vi "Write1000.vi"() -> ()   [LabVIEW 2015]
uses:
  <vilib>/Platform/TimedLoop/XDataNode/timing_clust.ctl
  <vilib>/Platform/TimedLoop/XDataNode/nitl_modes.ctl
  <vilib>/Platform/TimedLoop/XDataNode/wakeup.ctl
  <vilib>/platform/TimedLoop/XDataNode/XDataNode.xnode
  <vilib>/Platform/TimedLoop/XDataNode/XDNodeRunTimeDep.lvlib
panel:
  out "floor(x/y)":dbl
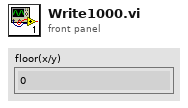
[diagram p1: front panel]
types:
  T1 = typedef "XDNodeRunTimeDep.lvlib/timing_clust.ctl" = cluster{"Expected End [f-1]":u64, "Actual End [f-1]":u64, "Finished Late? [f-1]":bool, "Expected End [i-1]":u64, "Actual End [i-1]":u64, "Finished Late? [i-1]":bool, "Expected Start [i]":u64, "Actual Start [i]":u64, "Expected Start [f]":u64, "Actual Start [f]":u64, "Source Name":string, "Structure Name":string, "Period":i64, "Deadline":i64, "Offset":i64, "Start":i64, "Priority":i32, "Timeout":i32, "Mode":T2, "Wakeup Reason":T3, "Error":errorcluster, "Source Type":string, "Secondary Source Type":string, "Global End Time":u64, "Global Start Time":u64, "Frame Duration":u64, "Iteration Duration":u64, "Assigned CPU":i32, "I/O Scan Engine Mode":u32}
  T2 = typedef "XDNodeRunTimeDep.lvlib/nitl_modes.ctl" = enum32{"No Change", "Process missed periods, maintain original phase", "Discard missed periods, maintain original phase", "Process missed periods, ignore original phase", "Discard missed periods, ignore original phase"}
  T3 = typedef "XDNodeRunTimeDep.lvlib/wakeup.ctl" = enum32{"Normal", "Aborted", "Asynchronous wakeup", "Timing source error", "Timed loop error", "Timeout"}
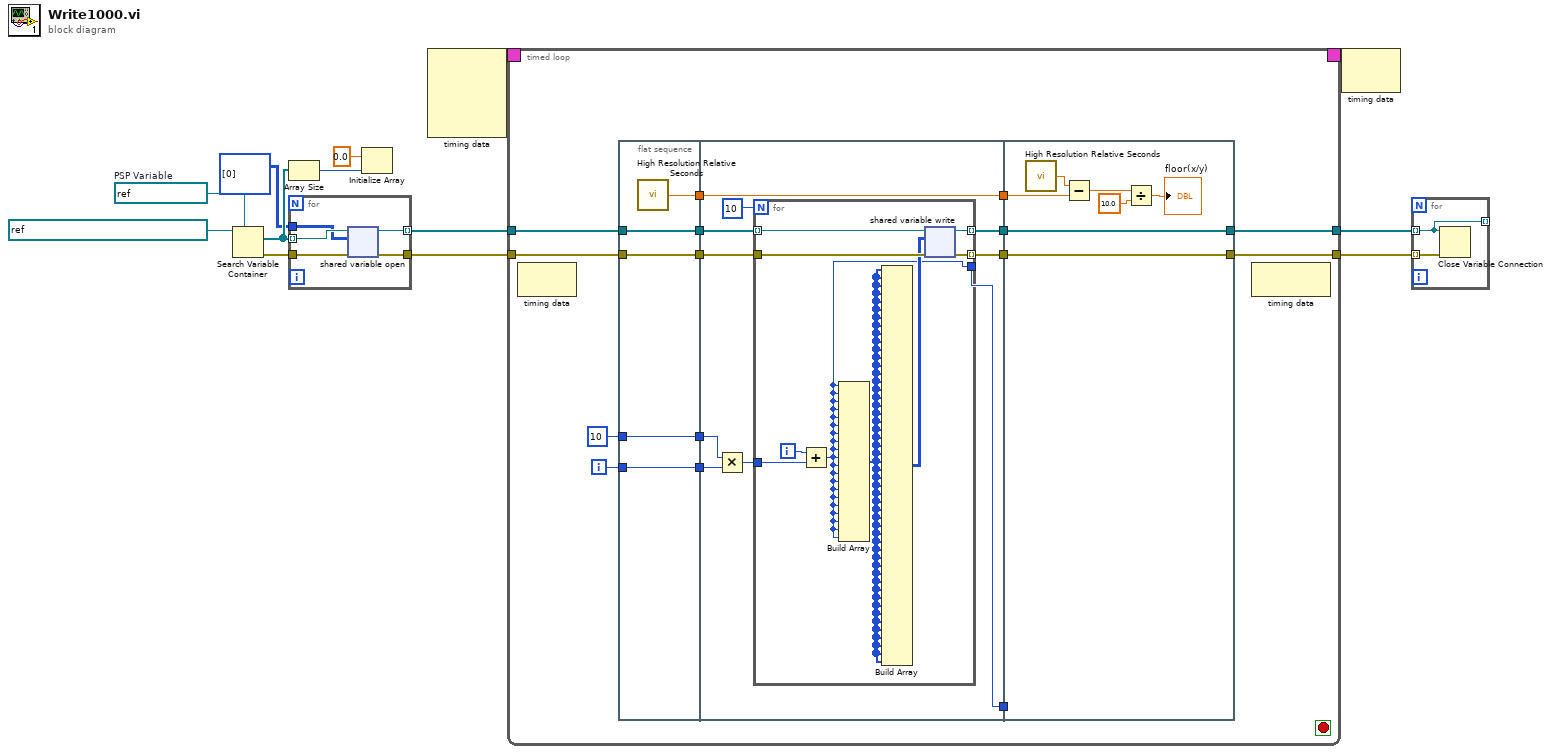
[diagram p0: block diagram]
diagram:
  w13 = refnum<k21> refnum  # PSP Variable
  n1 = Search Variable Container(7:w13, 11:refnum<k21> "ni.var.psp://localhost/Lib1000" ("container refnum in")) -> (0:w11:errorcluster, 2:w7:refnum<k21>[])  [unwired: 4 in, 1 out]
  n2 = Array Size(array=w7) -> (size(s)=w6:i32)
  n3 = for {
    tunnel: w7 -> [w18] mode=indexing
    tunnel: w11 -> [w17]
    tunnel: [w16] -> w3 mode=indexing
    tunnel: [w15] -> w8
    tunnel: i32[][] [[0]] ("appended array") -> [w14]
    n4 = shared-variable-open(w18, w17, w14) -> (w16:refnum<k21>, w15:errorcluster)  [unwired: 1 in]
  }
  n5 = Initialize Array(0.0 ("element"), w6) -> ()  [unwired: 1 out]
  n6 = node-c288() -> (w10:T1)  [unwired: 4 in]
  n7 = timed-loop {
    timing: w10 -> [_]
    timing-out: [_] -> w9
    tunnel: w3 -> [w33]
    tunnel: w8 -> [w32]
    tunnel: [w28] -> w4
    tunnel: [w29] -> w2
    i -> [w31]
    stop <- _ stop-if-true
    n8 = node-c288() -> ()  [unwired: 1 in, 1 out]
    n9 = flat-sequence {
      tunnel: 10 ("x") -> [w35]
      tunnel: w31 -> [w36]
      tunnel: w32 -> [w37]
      tunnel: w33 -> [w38]
      tunnel: [w38] -> w25
      tunnel: [w37] -> w24
      tunnel: [w36] -> w23
      tunnel: [w35] -> w22
      tunnel: [w34] -> w20
      tunnel: [w43] -> w27
      tunnel: [w42] -> w26
      tunnel: w25 -> [w48]
      tunnel: w24 -> [w47]
      tunnel: w23 -> [w46]
      tunnel: w22 -> [w45]
      tunnel: [w39] -> w21
      tunnel: w20 -> [w39]
      tunnel: [w41] -> w19
      tunnel: [w63] -> w28
      tunnel: [w64] -> w29
      tunnel: w27 -> [w64]
      tunnel: w26 -> [w63]
      tunnel: w21 -> [w61]
      tunnel: w19 -> [_]
      frame #0 {
        n10 = call <vilib>:"High Resolution Relative Seconds.vi"() -> ("relative seconds"=w34:dbl)
      }
      frame #1 {
        n11 = Multiply(x=w45, y=w46) -> (x*y=w44:i32)
        n12 = for {
          N: 10 -> [_]
          tunnel: w48 -> [w54] mode=indexing
          tunnel: w47 -> [w53]
          tunnel: w44 -> [w55]
          tunnel: [w51] -> w43 mode=indexing
          tunnel: [w50] -> w42 mode=indexing
          tunnel: [w49] -> w41
          i -> [w56]
          n13 = Add(x=w56, y=w55) -> (x+y=w49:i32)
          n14 = Build Array(w49, w49, w49, w49, w49, w49, w49, w49, w49, w49, w49, w49, w49, w49, w49, w49, w49, w49, w49, w49) -> (w57:i32[])
          n15 = Build Array(w57, w57, w57, w57, w57, w57, w57, w57, w57, w57, w57, w57, w57, w57, w57, w57, w57, w57, w57, w57, w57, w57, w57, w57, w57, w57, w57, w57, w57, w57, w57, w57, w57, w57, w57, w57, w57, w57, w57, w57, w57, w57, w57, w57, w57, w57, w57, w57, w57, w57) -> (w52:i32[][])
          n16 = shared-variable-write(w54, w53, w52) -> (w51:refnum<k21>, w50:errorcluster)
        }
      }
      frame #2 {
        n17 = call <vilib>:"High Resolution Relative Seconds.vi"() -> ("relative seconds"=w62:dbl)
        n18 = Subtract(x=w62, y=w61) -> (x-y=w60:dbl)
        n19 = Divide(x=w60, y=10.0) -> (x/y=→"floor(x/y)":dbl)
      }
    }
    n20 = node-c288() -> ()  [unwired: 1 in, 1 out]
  }
  n21 = node-c288(w9) -> ()  [unwired: 1 out]
  n22 = for {
    tunnel: w4 -> [w68] mode=indexing
    tunnel: [w67] -> _ mode=indexing
    tunnel: w2 -> [w67] mode=indexing
    n23 = Close Variable Connection(8:w68, 11:w67) -> ()  [unwired: 1 out]
  }
